vi "Init_Test.vi"() -> ()   [LabVIEW 2012]
panel:
  in  "ThorLabsPro8000":refnum<visa-resource-name>="COM3"
  out "ThorLabs Keys/Values":cluster{string, dbl}[](array[cluster])=[{"On TEC SLOT", 1.0}, {"On LD SLOT", 2.0}, {"Off TEC SLOT", 3.0}, {"Off LD SLOT", 4.0}, {"Etalon TEC SLOT", 5.0}, {"TSOA TEC SLOT", 6.0}, {"On Temp (C)", 19.86}, {"On P-const", 1.2}, {"On I-const", 1.2}, {"On D-const", 1.2}, {"On T-window", 1.0}, {"On TempSens", 1.0}, {"On Current (mA)", 139.5}, {"On Polarity", 1.0}, {"On TP-SLOT", 1.0}, {"On TP", 1.0}, {"Off Temp (C)", 17.47}, {"Off P-const", 1.2}, {"Off I-const", 1.2}, {"Off D-const", 1.2}, {"Off T-window", 1.0}, {"Off TempSens", 1.0}, {"Off Current (mA)", 148.5}, {"Off Polarity", 1.0}, {"Off TP-SLOT", 3.0}, {"Off TP", 1.0}, {"Etalon Temp (C)", 26.14}, {"Etalon P-const", 50.0}, {"Etalon I-const", 2.0}, {"Etalon D-const", 2.0}, {"Etalon T-window", 1.0}, {"Etalon TempSens", 0.0}, {"TSOA Temp (C)", 18.0}, {"TSOA P-const", 1.2}, {"TSOA I-const", 1.2}, {"TSOA D-const", 1.2}, {"TSOA T-window", 1.0}, {"TSOA TempSens", 1.0}, {"Warm-up Time (s)", 30.0}]
  out "Keys Not Found":string[](array[string])
  out "Missing Key Value":bool
  out "All Keys Found":bool
  in  "Init File Name":path=path "C:/LabVIEW_2014/H2O_DIAL/h2o_dial_settings-2.txt"
  in  "Error In":errorcluster caption="error in"
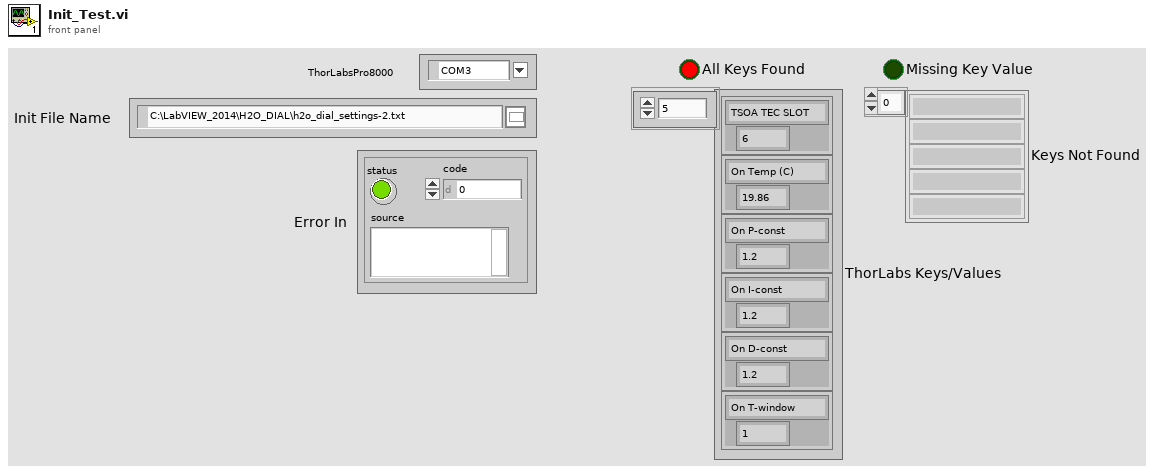
[diagram p1: front panel]
types:
  T1 = cluster{"String":string, "Numeric Indicator":dbl}[]
  T2 = typedef "ThorLabsCluster.ctl" = cluster{"OnTecSlot":dbl, "OnLdSlot":dbl, "OnTemp":dbl, "OnCurrent":dbl, "OnLimit":dbl, "OnLDMode":dbl, "OnPconst":dbl, "OnIconst":dbl, "OnDconst":dbl, "OnTpSlot":dbl, "OnTp":dbl, "OnPolarity":dbl, "OnTempSens":dbl, "OnTwindow":dbl, "OffTecSlot":dbl, "OffLdSlot":dbl, "OffTemp":dbl, "OffCurrent":dbl, "OnffLimit":dbl, "OffLDMode":dbl, "OffPconst":dbl, "OffIconst":dbl, "OffDconst":dbl, "OffTpSlot":dbl, "OffTp":dbl, "OffPolarity":dbl, "OffTempSens":dbl, "OffTwindow":dbl, "EtalonTecSlot":dbl, "EtalonTemp":dbl, "EtalonPconst":dbl, "EtalonIconst":dbl, "EtalonDconst":dbl, "EtalonTempSens":dbl, "EtalonTwindow":dbl, "TosaTecSlot":dbl, "TosaTemp":dbl, "TosaPconst":dbl, "TosaIconst":dbl, "TosaDconst":dbl, "TosaTempSens":dbl, "TosaTwindow":dbl, "WarmUpTime":dbl}
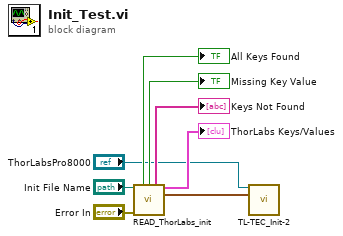
[diagram p0: block diagram]
diagram:
  n1 = call "READ_ThorLabs_init.vi"("Init File Name"="Init File Name", "Error In"="Error In") -> ("All Keys Found"=→"All Keys Found":bool, "Missing Key Value"=→"Missing Key Value":bool, "Keys Not Found"=→"Keys Not Found":string[], "Init Keywords and Values"=→"ThorLabs Keys/Values":T1, "ThorLabsCluster"=w2:T2)  [unwired: 8 in, 1 out]
  n2 = call "TL-TEC_Init-2.vi"("ThorLabsPro8000"="ThorLabsPro8000", "ThorLabsCluster"=w2) -> ()  [unwired: 13 in, 1 out]
